vi "Write Child Attributes.vi"(10 "Child Attributes":T1, 11 "Actor in":refnum<class "Actor.lvclass">) -> (3 "Actor out":refnum<class "Actor.lvclass">)   [LabVIEW 2020, in "jettl.lvlib" / "Actor.lvclass"]
uses:
  Actor.lvclass
  Msg/Msg.lvclass
  Transport/Transport.lvclass
  Attributes Metadata/Attributes Metadata.lvclass
  Child Attributes.ctl
  jettl.lvlib
  Msgs.ctl
  Attributes.ctl
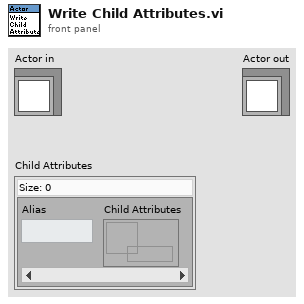
[diagram p1: front panel]
types:
  T1 = typedef "jettl.lvlib/Child Attributes.ctl" = map{string, refnum<data-value>}
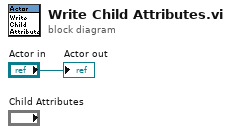
[diagram p0: block diagram]
diagram:
  "Actor out" <- "Actor in"
